vi "Data to host.vi"(8 "error in":errorcluster, 11 "Queue ref":T1) -> (0 "error out":errorcluster, 3 "data to Host":string)   [LabVIEW 2022 SP3]
uses:
  RT Controls/RT All Queue.ctl
  RT Controls/RT All Loop Status.ctl
  RT Controls/DO FGV.ctl
  RT Controls/AO FGV.ctl
  RT Global.vi
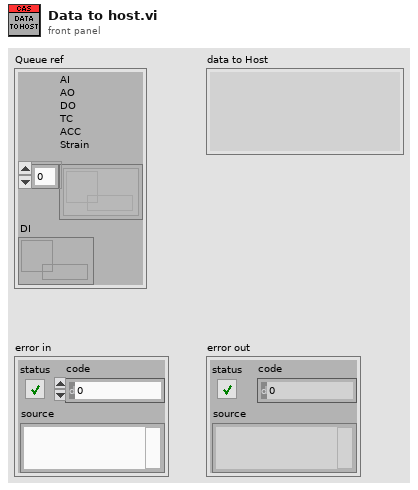
[diagram p1: front panel]
types:
  T1 = typedef "RT All Queue.ctl" = cluster{"AI\nAO\nDO\nTC\nACC\nStrain":refnum<queue>[], "DI":refnum<queue>}
  T2 = enum16{"Init", "Read 'All'", "Read 'n'", "Read '1'", "Write '1'", "Write 'n'", "Write 'All'"}
  T3 = cluster{"AI Data":waveform(dbl)[], "AO Data":waveform(dbl)[], "DO Data":waveform(dbl)[], "TC Data":waveform(dbl)[], "ACC Data":waveform(dbl)[], "Strain Data":waveform(dbl)[], "DI Data":digitalwaveform[], "All Status":bool[], "Channel List":cluster{"AI Channel list":tag[], "AO Channel list":tag[], "DO Channel list ":tag[], "DI Channel list":tag[]}, "ALS DO":bool[], "ALS AO":dbl[], "Seq State":string}
  T4 = typedef "AO FGV.ctl" = enum16{"Read", "Write", "Start time", "init", "Read Only"}
  T5 = typedef "DO FGV.ctl" = enum16{"Read", "Write", "Start time", "init", "Read only"}
  T6 = typedef "RT All Loop Status.ctl" = enum16{"AI", "AO", "DI", "DO", "TC", "Strain", "ACC", "RT", "Log", "Seq", "Sync"}
  T7 = cluster{"AI Channel list":tag[], "AO Channel list":tag[], "DO Channel list ":tag[], "DI Channel list":tag[]}
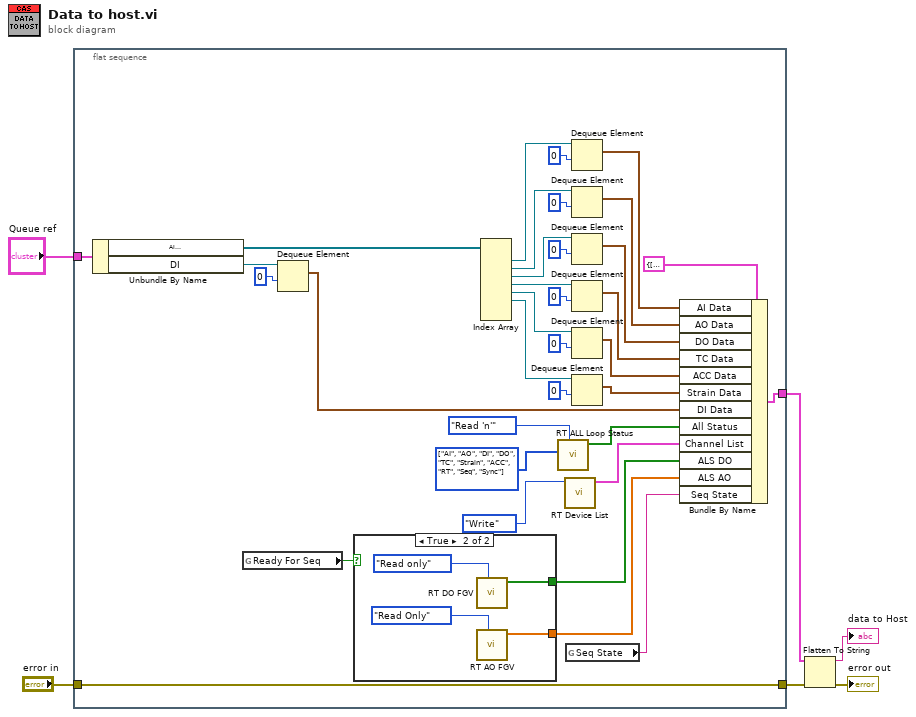
[diagram p0: block diagram]
diagram:
  n1 = flat-sequence {
    tunnel: "Queue ref" -> [w41]
    tunnel: [w18] -> w4
    tunnel: "error in" -> [w11]
    tunnel: [w11] -> w2
    frame #0 {
      w14 = T6[] [enum."AI", enum."AO", enum."DI", enum."DO", enum."TC", enum."Strain", enum."ACC", enum."RT", enum."Seq", enum."Sync"] items=["AI", "AO", "DI", "DO", "TC", "Strain", "ACC", "RT", "Log", "Seq", "Sync"] ("Loops")
      n2 = Unbundle By Name(w41) -> ("AI\nAO\nDO\nTC\nACC\nStrain"=w40:refnum<queue>[], "DI"=w27:refnum<queue>)
      n3 = global read "RT Global.vi" "Ready For Seq"() -> (w9:bool)
      n4 = Dequeue Element(queue=w27, timeout in ms (-1)=0) -> (element=w19:digitalwaveform[])  [unwired: 1 in, 3 out]
      n5 = case shown="True" w9 {
        tunnel: [_ w45] -> w10
        tunnel: [_ w42] -> w8
        frame False {
        }
        frame True {
          n6 = call "RT DO FGV.vi"("Enum"=DO_FGV."Read only") -> ("DO out"=w45:bool[])  [unwired: 8 in, 2 out]
          n7 = call "RT AO FGV.vi"("Enum"=AO_FGV."Read Only") -> ("AO out"=w42:dbl[])  [unwired: 8 in, 2 out]
        }
      }
      n8 = Index Array(array=w40) -> (element #1=w39:refnum<queue>, element #2=w38:refnum<queue>, element #3=w37:refnum<queue>, element #4=w36:refnum<queue>, element #5=w35:refnum<queue>, element #6=w34:refnum<queue>)  [unwired: 8 in, 2 out]
      n9 = call "RT ALL Loop Status.vi"("Option"=T2."Read 'n'", "Loops"=w14) -> ("Status List Out"=w16:bool[])  [unwired: 7 in, 2 out]
      n10 = call "RT Device List.vi"("Enum"=enum16{"Read", "Write"}."Write") -> ("Channel List"=w12:T7)  [unwired: 8 in, 1 out]
      n11 = global read "RT Global.vi" "Seq State"() -> (w7:string)
      n12 = Dequeue Element(queue=w39, timeout in ms (-1)=0) -> (element=w25:waveform(dbl)[])  [unwired: 1 in, 3 out]
      n13 = Dequeue Element(queue=w38, timeout in ms (-1)=0) -> (element=w24:waveform(dbl)[])  [unwired: 1 in, 3 out]
      n14 = Dequeue Element(queue=w37, timeout in ms (-1)=0) -> (element=w23:waveform(dbl)[])  [unwired: 1 in, 3 out]
      n15 = Dequeue Element(queue=w36, timeout in ms (-1)=0) -> (element=w22:waveform(dbl)[])  [unwired: 1 in, 3 out]
      n16 = Dequeue Element(queue=w35, timeout in ms (-1)=0) -> (element=w21:waveform(dbl)[])  [unwired: 1 in, 3 out]
      n17 = Dequeue Element(queue=w34, timeout in ms (-1)=0) -> (element=w20:waveform(dbl)[])  [unwired: 1 in, 3 out]
      n18 = Bundle By Name(cluster=T3 {"AI Data"=[], "AO Data"=[], "DO Data"=[], "TC Data"=[], "ACC Data"=[], "Strain Data"=[], "DI Data"=[], "All Status"=[], "Channel List"={"AI Channel list"=[], "AO Channel list"=[], "DO Channel list "=[], "DI Channel list"=[]}, "ALS DO"=[], "ALS AO"=[], "Seq State"=""}, "AI Data"=w25, "AO Data"=w24, "DO Data"=w23, "TC Data"=w22, "ACC Data"=w21, "Strain Data"=w20, "DI Data"=w19, "All Status"=w16, "Channel List"=w12, "ALS DO"=w10, "ALS AO"=w8, "Seq State"=w7) -> (w18:T3)
    }
  }
  n19 = Flatten To String(anything=w4, error in (no error)=w2) -> (data string=→"data to Host":string, error out=→"error out":errorcluster)  [unwired: 2 in, 1 out]
